vi "DAQ signal generation vi.vi"(6 "Time for each step":dbl, 9 "Total time":dbl, 10 "DAQ 1":waveform(dbl)[](array[waveform]), 11 "DAQ 2":waveform(dbl)[](array[waveform])) -> (0 "error out":errorcluster, 3 "error out 7":errorcluster)   [LabVIEW 2016]
uses:
  <vilib>/DAQmx/write.llb/DAQmx Write (Analog 1D Wfm NChan NSamp).vi
  <vilib>/DAQmx/create/channels.llb/DAQmx Create Channel (AO-Voltage-Basic).vi
  <vilib>/DAQmx/configure/timing.llb/DAQmx Timing (Sample Clock).vi
  <vilib>/DAQmx/miscellaneous.llb/DAQmx Fill In Error Info.vi
  <vilib>/DAQmx/configure/trigger.llb/DAQmx Start Trigger (Digital Edge).vi
  <resource>/objmgr/daqmx.rc
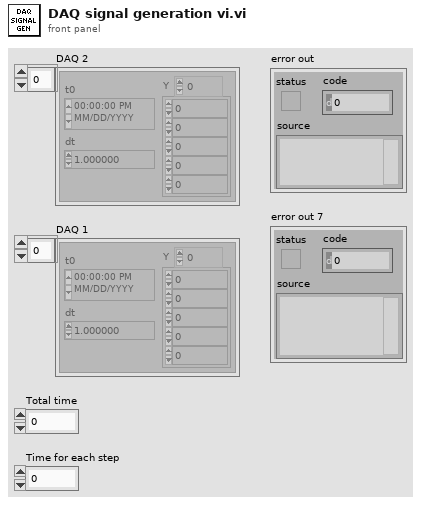
[diagram p1: front panel]
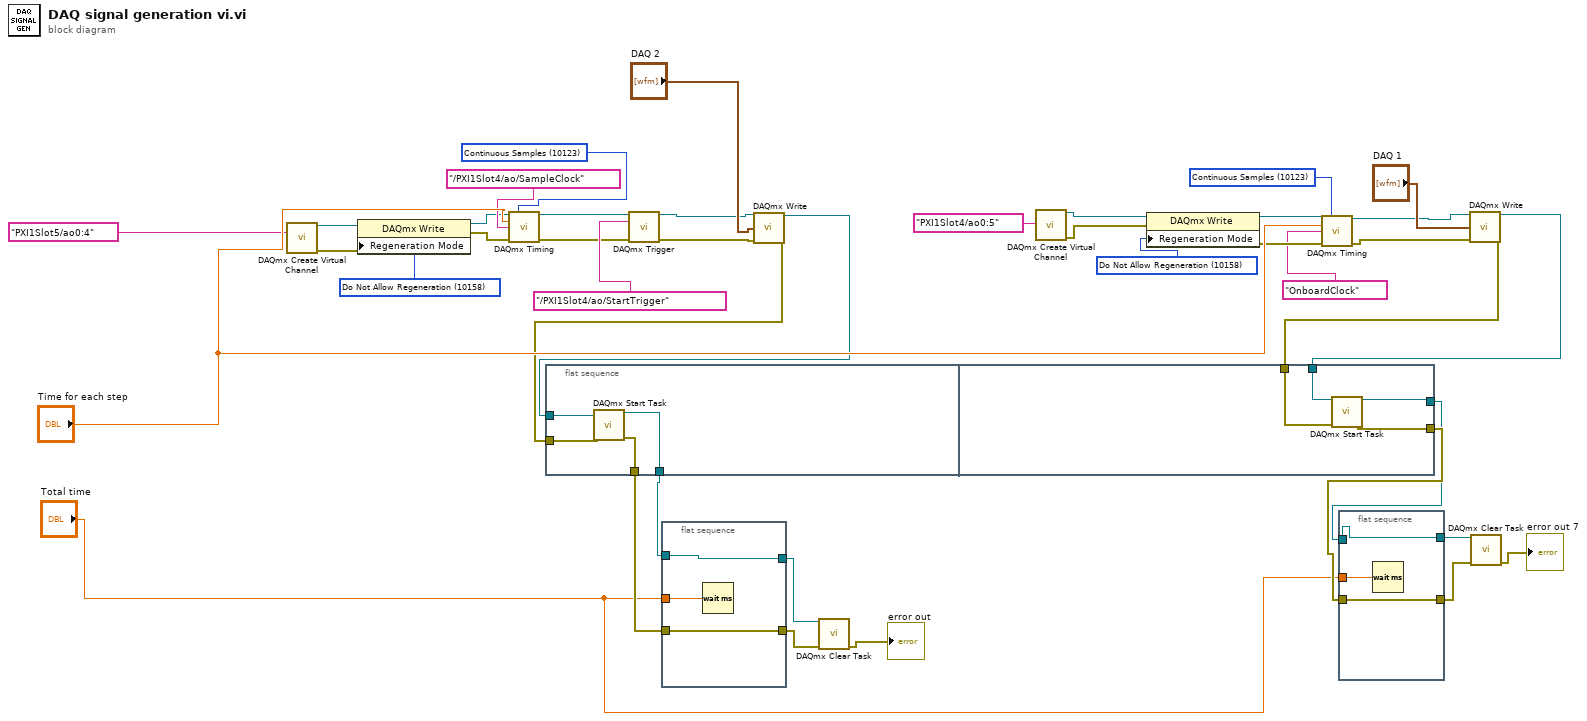
[diagram p0: block diagram]
diagram:
  w38 = 10158 items=["Allow Regeneration"=10097, "Do Not Allow Regeneration"=10158] ("RegenMode")
  w20 = 10158 items=["Allow Regeneration"=10097, "Do Not Allow Regeneration"=10158] ("RegenMode")
  w19 = 10123 items=["Finite Samples"=10178, "Continuous Samples"=10123, "Hardware Timed Single Point"=12522] ("sample mode")
  w13 = 10123 items=["Finite Samples"=10178, "Continuous Samples"=10123, "Hardware Timed Single Point"=12522] ("sample mode")
  n1 = call-poly <vilib>:"DAQmx Create Virtual Channel.vi"("physical channels"=tag "PXI1Slot5/ao0:4") -> ("task out"=w15:refnum<k21>, "error out"=w16:errorcluster)  [unwired: 13 in]
  n2 = property class="DAQmx Write"(reference=w15, error in=w16, "Regeneration Mode"=w20) -> (reference out=w17:refnum<k21>, error out=w18:errorcluster)
  n3 = call-poly <vilib>:"DAQmx Timing.vi"("task/channels in"=w17, "sample mode"=w19, "rate"="Time for each step", "source"=tag "/PXI1Slot4/ao/SampleClock", "error in"=w18) -> ("task out"=w21:refnum<k21>, "error out"=w22:errorcluster)  [unwired: 9 in]
  n4 = flat-sequence {
    tunnel: w26 -> [w45]
    tunnel: w27 -> [w44]
    tunnel: [w43] -> w6
    tunnel: [w42] -> w8
    tunnel: w31 -> [w49]
    tunnel: w32 -> [w48]
    tunnel: [w46] -> w2
    tunnel: [w47] -> w3
    frame #0 {
      n5 = call <vilib>:"DAQmx Start Task.vi"("task/channels in"=w44, "error in"=w45) -> ("task out"=w42:refnum<k21>, "error out"=w43:errorcluster)  [unwired: 12 in]
    }
    frame #1 {
      n6 = call <vilib>:"DAQmx Start Task.vi"("task/channels in"=w49, "error in"=w48) -> ("task out"=w46:refnum<k21>, "error out"=w47:errorcluster)  [unwired: 12 in]
    }
  }
  n7 = call-poly <vilib>:"DAQmx Trigger.vi"("task/channels in"=w21, "source"=tag "/PXI1Slot4/ao/StartTrigger", "error in"=w22) -> ("task out"=w28:refnum<k21>, "error out"=w29:errorcluster)  [unwired: 11 in]
  n8 = flat-sequence {
    tunnel: [w52] -> w9
    tunnel: w8 -> [w52]
    tunnel: [w51] -> w7
    tunnel: w6 -> [w51]
    tunnel: "Total time" -> [w50]
    frame #0 {
      n9 = Wait (ms)(milliseconds to wait=w50) -> ()  [unwired: 1 out]
    }
  }
  n10 = call-poly <vilib>:"DAQmx Write.vi"("task/channels in"=w28, "data"="DAQ 2", "error in"=w29) -> ("task out"=w27:refnum<k21>, "error out"=w26:errorcluster)  [unwired: 10 in, 1 out]
  n11 = call <vilib>:"DAQmx Clear Task.vi"("task in"=w9, "error in"=w7) -> ("error out"=→"error out":errorcluster)  [unwired: 13 in]
  n12 = call-poly <vilib>:"DAQmx Create Virtual Channel.vi"("physical channels"=tag "PXI1Slot4/ao0:5") -> ("task out"=w36:refnum<k21>, "error out"=w37:errorcluster)  [unwired: 13 in]
  n13 = property class="DAQmx Write"(reference=w36, error in=w37, "Regeneration Mode"=w38) -> (reference out=w34:refnum<k21>, error out=w35:errorcluster)
  n14 = call-poly <vilib>:"DAQmx Timing.vi"("task/channels in"=w34, "sample mode"=w13, "rate"="Time for each step", "source"=tag "OnboardClock", "error in"=w35) -> ("task out"=w14:refnum<k21>, "error out"=w33:errorcluster)  [unwired: 9 in]
  n15 = flat-sequence {
    tunnel: [w55] -> w5
    tunnel: w2 -> [w55]
    tunnel: [w54] -> w4
    tunnel: w3 -> [w54]
    tunnel: "Total time" -> [w53]
    frame #0 {
      n16 = Wait (ms)(milliseconds to wait=w53) -> ()  [unwired: 1 out]
    }
  }
  n17 = call-poly <vilib>:"DAQmx Write.vi"("task/channels in"=w14, "data"="DAQ 1", "error in"=w33) -> ("task out"=w31:refnum<k21>, "error out"=w32:errorcluster)  [unwired: 10 in, 1 out]
  n18 = call <vilib>:"DAQmx Clear Task.vi"("task in"=w5, "error in"=w4) -> ("error out"=→"error out 7":errorcluster)  [unwired: 13 in]
